vi "Get SMO PGSQL Log Paths.vi"(8 "error in (no error)":errorcluster, 11 "RP100 in":refnum<class "RP100.lvclass">) -> (0 "error out":errorcluster, 2 "Paths":string, 3 "RP100 out":refnum<class "RP100.lvclass">)   [LabVIEW 2019, in "RP100.lvclass"]
uses:
  RP100.lvclass
  <userlib>/LevyLab/Levylab Instruments/Instrument Types/Strain/Instrument.Strain.lvclass
  Typedefs/getAll.ctl
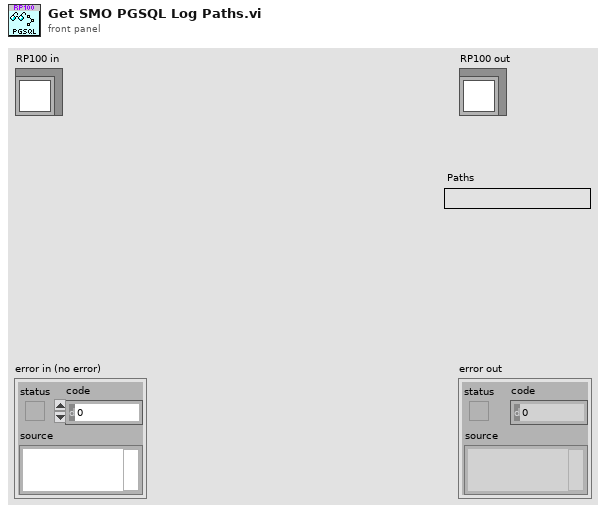
[diagram p1: front panel]
types:
  T1 = typedef "RP100.lvclass/getAll.ctl" = cluster{"Output State Ch1":string, "Output State Ch2":string, "Level (V) Ch1":dbl, "Level (V) Ch2":dbl, "Slew (V/s) Ch1":dbl, "Slew (V/s) Ch2":dbl, "measured V Ch1":dbl, "measured V Ch2":dbl, "measured I Ch1":dbl, "measured I Ch2":dbl}
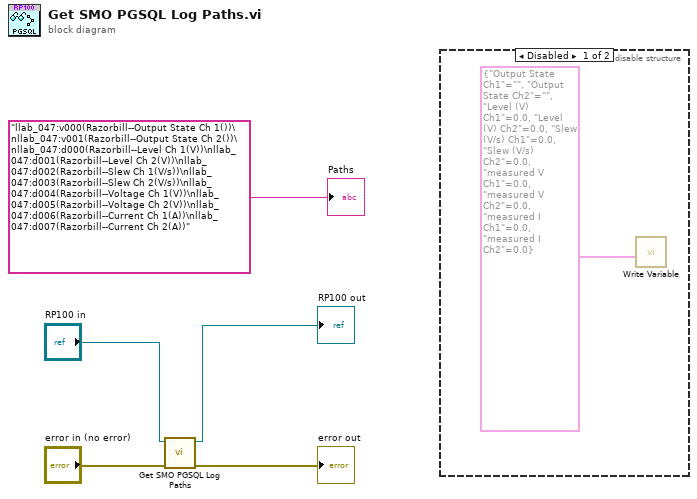
[diagram p0: block diagram]
diagram:
  n1 = call-parent "Get SMO PGSQL Log Paths.vi"("error in (no error)"="error in (no error)", "Instrument in"="RP100 in") -> ("error out"=→"error out":errorcluster, "Instrument out"=→"RP100 out":refnum<class "RP100.lvclass">)  [unwired: 7 in, 1 out]
  n2 = disable-structure shown="Disabled" {
    frame Disabled {
      n3 = call <userlib>:"Write Variable.vi"("Data"=T1 {"Output State Ch1"="", "Output State Ch2"="", "Level (V) Ch1"=0.0, "Level (V) Ch2"=0.0, "Slew (V/s) Ch1"=0.0, "Slew (V/s) Ch2"=0.0, "measured V Ch1"=0.0, "measured V Ch2"=0.0, "measured I Ch1"=0.0, "measured I Ch2"=0.0} ("Cluster")) -> ()  [unwired: 8 in, 3 out]
    }
    frame Enabled {
    }
  }
  "Paths" <- "llab_047:v000(Razorbill--Output State Ch 1())\nllab_047:v001(Razorbill--Output State Ch 2())\nllab_047:d000(Razorbill--Level Ch 1(V))\nllab_047:d001(Razorbill--Level Ch 2(V))\nllab_047:d002(Razorbill--Slew Ch 1(V/s))\nllab_047:d003(Razorbill--Slew Ch 2(V/s))\nllab_047:d004(Razorbill--Voltage Ch 1(V))\nllab_047:d005(Razorbill--Voltage Ch 2(V))\nllab_047:d006(Razorbill--Current Ch 1(A))\nllab_047:d007(Razorbill--Current Ch 2(A))" ("Paths")
